vi "Simulator PFE Config Test.vi"(4 "error in (no error)":errorcluster, 6 "Configuration":T1={"BusType"=enum."PCI/ISA/PCMCIA", "Card"=0, "USB"=0, "IP"=1, "COM"=1, "Baud Rate"=enum."9600"}, 7 "Str Refnum":refnum<vi>) -> (0 "error out":errorcluster)   [LabVIEW 2011]
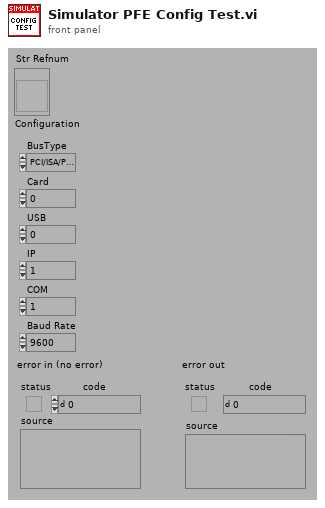
[diagram p1: front panel]
types:
  T1 = cluster{"BusType":enum32{"PCI/ISA/PCMCIA", "USB", "Ethernet", "Serial"}, "Card":i32, "USB":i32, "IP":u32, "COM":i32, "Baud Rate":enum16{"300", "600", "1200", "2400", "4800", "9600"}}
  T2 = enum32{"PCI/ISA/PCMCIA", "USB", "Ethernet", "Serial"}
  T3 = enum16{"300", "600", "1200", "2400", "4800", "9600"}
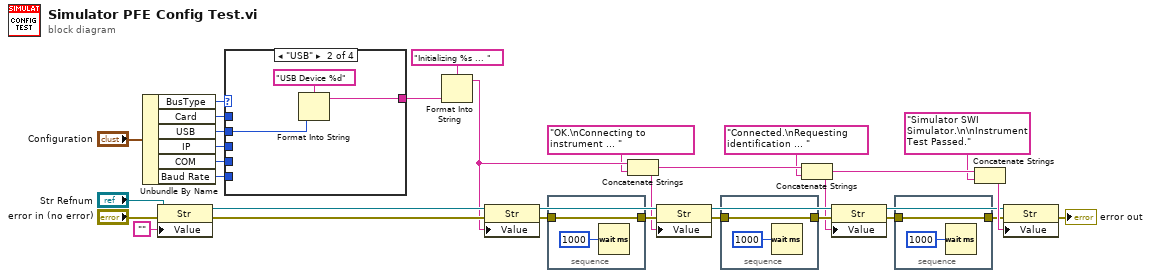
[diagram p0: block diagram]
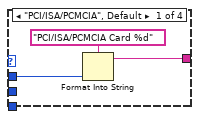
[diagram p2: hidden frame]
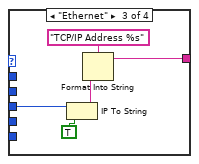
[diagram p3: hidden frame]
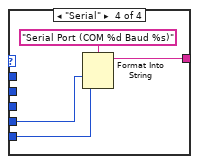
[diagram p4: hidden frame]
diagram:
  n1 = Unbundle By Name("Configuration") -> ("BusType"=w25:T2, "Card"=w24:i32, "USB"=w23:i32, "IP"=w22:u32, "COM"=w21:i32, "Baud Rate"=w1:T3)
  n2 = property class="Str"(reference="Str Refnum", error in="error in (no error)", "Value"="") -> (reference out=w18:refnum<vi>, error out=w28:errorcluster)
  n3 = case shown="\"USB\"" w25 {
    tunnel: w24 -> [w33 _ _ _]
    tunnel: w23 -> [_ w35 _ _]
    tunnel: w22 -> [_ _ w41 _]
    tunnel: w21 -> [_ _ _ w45]
    tunnel: [w32 w36 w38 w44] -> w20
    tunnel: w1 -> [_ _ _ w43]
    frame "PCI/ISA/PCMCIA", Default {
      n4 = Format Into String(format string="PCI/ISA/PCMCIA Card %d", w33) -> (resulting string=w32:string)  [unwired: 2 in, 1 out]
    }
    frame "USB" {
      n5 = Format Into String(format string="USB Device %d", w35) -> (resulting string=w36:string)  [unwired: 2 in, 1 out]
    }
    frame "Ethernet" {
      n6 = IP To String(1:TRUE, 2:w41) -> (0:w40:string)
      n7 = Format Into String(format string="TCP/IP Address %s", w40) -> (resulting string=w38:string)  [unwired: 2 in, 1 out]
    }
    frame "Serial" {
      n8 = Format Into String(format string="Serial Port (COM %d Baud %s)", w45, w43) -> (resulting string=w44:string)  [unwired: 2 in, 1 out]
    }
  }
  n9 = Format Into String(format string="Initializing %s ... ", w20) -> (resulting string=w11:string)  [unwired: 2 in, 1 out]
  n10 = property class="Str"(reference=w18, error in=w28, "Value"=w11) -> (reference out=w16:refnum<vi>, error out=w19:errorcluster)
  n11 = stacked-sequence {
    tunnel: w19 -> [w47]
    tunnel: [w47] -> w17
    frame #0 {
      n12 = Wait (ms)(milliseconds to wait=u32 1000) -> ()  [unwired: 1 out]
    }
  }
  n13 = Concatenate Strings(w11, "OK.\nConnecting to instrument ... ") -> (w9:string)
  n14 = property class="Str"(reference=w16, error in=w17, "Value"=w9) -> (reference out=w13:refnum<vi>, error out=w15:errorcluster)
  n15 = stacked-sequence {
    tunnel: w15 -> [w49]
    tunnel: [w49] -> w14
    frame #0 {
      n16 = Wait (ms)(milliseconds to wait=u32 1000) -> ()  [unwired: 1 out]
    }
  }
  n17 = Concatenate Strings(w9, "Connected.\nRequesting identification ... ") -> (w5:string)
  n18 = property class="Str"(reference=w13, error in=w14, "Value"=w5) -> (reference out=w2:refnum<vi>, error out=w12:errorcluster)
  n19 = stacked-sequence {
    tunnel: w12 -> [w51]
    tunnel: [w51] -> w6
    frame #0 {
      n20 = Wait (ms)(milliseconds to wait=u32 1000) -> ()  [unwired: 1 out]
    }
  }
  n21 = Concatenate Strings(w5, "Simulator SWI Simulator.\n\nInstrument Test Passed.") -> (w7:string)
  n22 = property class="Str"(reference=w2, error in=w6, "Value"=w7) -> (error out=→"error out":errorcluster)  [unwired: 1 out]
